vi "Read IO 集合.vi"() -> (3 "IO集合":bool[](array[boolean]))   [LabVIEW 2017]
uses:
  Component Assemble Input.ctl
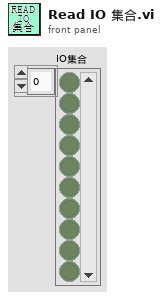
[diagram p1: front panel]
types:
  T1 = typedef "Component Assemble Input.ctl" = cluster{"Component Name":string, "Component State":bool, "D Value":i32}
  T2 = typedef "MX操作选项.ctl" = enum16{"MX Initial ", "MX Close", "X&Y&M Read", "X&Y&M Write", "D Read", "D Write", "Many component Read", "Many component Write", "Load Function Global"}
  T3 = typedef "State Assemble.ctl" = cluster{"Read State":bool, "Group State":bool[], "D值":i32}
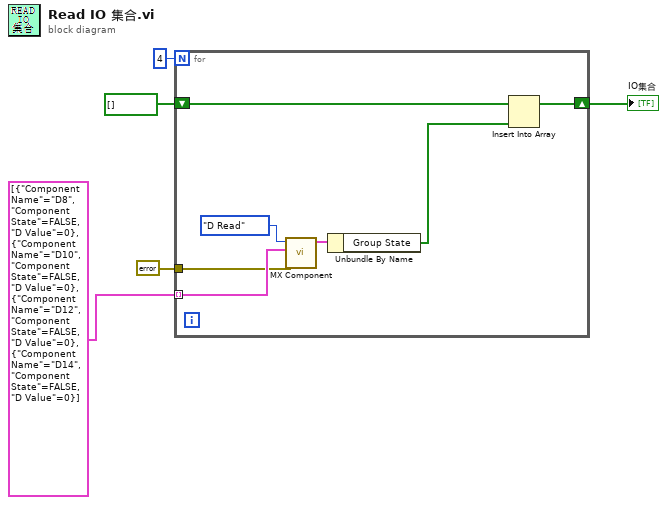
[diagram p0: block diagram]
diagram:
  n1 = for {
    N: 4 -> [_]
    tunnel: T1[] [{"Component Name"="D8", "Component State"=FALSE, "D Value"=0}, {"Component Name"="D10", "Component State"=FALSE, "D Value"=0}, {"Component Name"="D12", "Component State"=FALSE, "D Value"=0}, {"Component Name"="D14", "Component State"=FALSE, "D Value"=0}] -> [w11] mode=indexing
    tunnel: errorcluster {"status"=FALSE, "code"=0, "source"=""} ("错误输入") -> [w10]
    shift-right: [w6] -> w1
    shift-left: bool[] [] -> [w8]
    n2 = call "MX Component.vi"("错误输入"=w10, "Component Assemble Input"=w11, "MX操作选项"=MX操作选项."D Read") -> ("State Assemble"=w9:T3)  [unwired: 6 in, 2 out]
    n3 = Unbundle By Name(w9) -> ("Group State"=w7:bool[])
    n4 = Insert Into Array(array=w8, new element=w7) -> (w6:bool[])  [unwired: 1 in]
  }
  "IO集合" <- w1
